vi "Test Process Multiple Stop.vi"(8 "error in (no error)":errorcluster, 11 "Process Test In":refnum<class "Process Dev Test.lvclass">) -> (0 "error out":errorcluster, 3 "Process Test Out":refnum<class "Process Dev Test.lvclass">)   [LabVIEW 2020, in "Process Dev Test.lvclass"]
uses:
  Process Dev Test.lvclass
  C:/Program Files (x86)/National Instruments/LabVIEW 2020/vi.lib/Astemes/LUnit/Test Case.lvclass
  source/Framework Test Suite/Mock Error Handler/Mock Error Handler.lvclass
  C:/Git/astemes-triarc-framework/source/Framework/Error Handler Interface/Error Handler Interface.lvclass
  source/Framework/Process/Process.lvclass/Process.ctl
  <vilib>/Astemes/LUnit/Test Case.lvclass/Test Case.ctl
  <vilib>/Astemes/LUnit/LUnit Assertion Result.lvclass/LUnit Assertion Result.ctl
  <vilib>/Astemes/LUnit/LUnit Test Case Result.lvclass/LUnit Test Case Result.ctl
  <vilib>/Astemes/LUnit/LUnit Method Result.lvclass/LUnit Method Result.ctl
  source/Framework/Process/Protected/Messaging/Enqueue Message.vi
  source/Framework/Process/Public/Lifecycle/Get Lifecycle State.vi
  source/Framework/Process/Private/SubVIs/Wait for finish.vi
  source/Framework/Process/Private/SubVIs/Set Lifecycle State.vi
  <vilib>/Astemes/LUnit/Palette/Pass.vi
  <vilib>/Astemes/LUnit/Palette/Fail.vi
  <vilib>/Astemes/LUnit/Set Assertion Type.vi
  source/Framework/Process/Private/SubVIs/Handle Debug Data.vi
  <vilib>/Utility/error.llb/Clear Errors.vi
  <vilib>/Astemes/LUnit/Add test result.vi
  <vilib>/Astemes/LUnit/LUnit Write Passed.vi
  <vilib>/Astemes/LUnit/LUnit Write Message.vi
  <vilib>/Astemes/LUnit/LUnit Write Description.vi
  <vilib>/Astemes/LUnit/LUnit Write Assertion Type.vi
  source/Framework/Logging/Log Debug.vi
  <vilib>/AdvancedString/1D String Array to Delimited String.vi
  <vilib>/Utility/High Resolution Relative Seconds.vi
  <vilib>/Astemes/LUnit/LUnit Record Assertion Result.vi
  <vilib>/Astemes/LUnit/LUnit Aggregate Assertion Results.vi
  <vilib>/Astemes/LUnit/Assertion Result/LUnit Read Status.vi
  <vilib>/Astemes/LUnit/LUnit Read Message.vi
  <vilib>/Astemes/LUnit/LUnit Read Description.vi
  <vilib>/Astemes/LUnit/Method Result/LUnit Merge Status.vi
  <vilib>/Astemes/LUnit/LUnit Concatenate result strings.vi
  <vilib>/Utility/error.llb/Error Cluster From Error Code.vi
  source/Framework/Process/Public/Read Name.vi
  <vilib>/Astemes/LUnit/LUnit Assertion Result.lvclass
  source/Framework/Process/Process.lvclass
  <vilib>/Astemes/LUnit/Test Case.lvclass
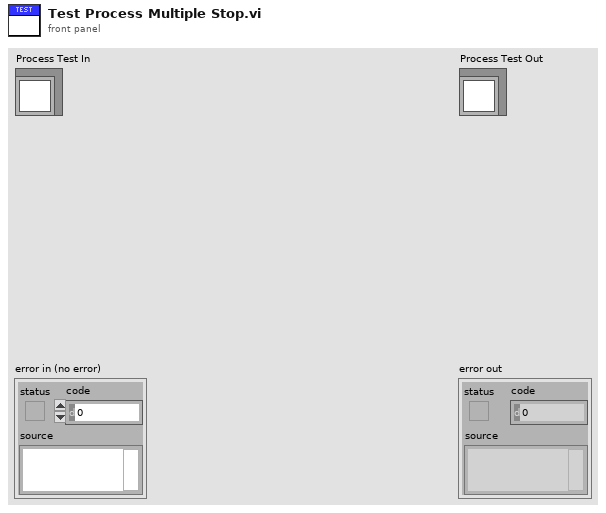
[diagram p1: front panel]
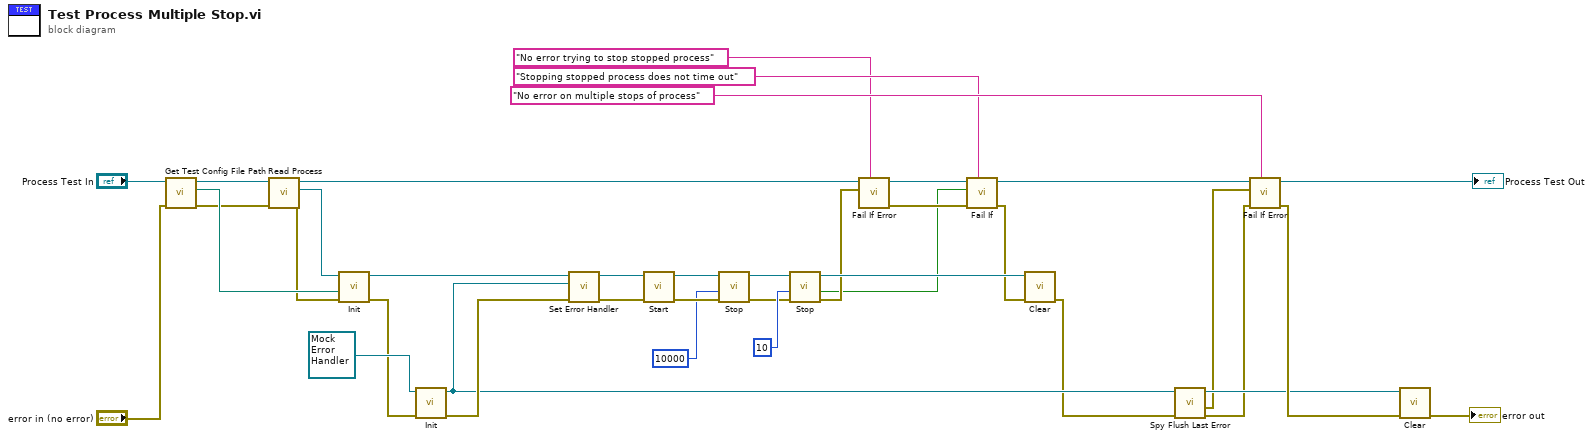
[diagram p0: block diagram]
diagram:
  n1 = call "Get Test Config File Path.vi"("error in (no error)"="error in (no error)", "Process Test In"="Process Test In") -> ("error out"=w29:errorcluster, "Test config path"=w32:path, "Process Test Out"=w34:refnum<class "Process Dev Test.lvclass">)  [unwired: 7 in]
  n2 = call "Read Process.vi"("error in (no error)"=w29, "Process Test in"=w34) -> ("error out"=w30:errorcluster, "Process.lvclass"=w31:refnum<class "Process.lvclass">, "Process Test out"=w10:refnum<class "Process Dev Test.lvclass">)  [unwired: 7 in]
  n3 = call-dynamic "Init.vi"("error in (no error)"=w30, "Config File Path"=w32, "Process In"=w31) -> ("error out"=w20:errorcluster, "Process Out"=w35:refnum<class "Process.lvclass">)  [unwired: 7 in]
  n4 = call-dynamic "Init.vi"("error in (no error)"=w20, "Mock Error Handler In"=refnum<class "Mock Error Handler.lvclass"> refnum ("Mock Error Handler.lvclass")) -> ("error out"=w24:errorcluster, "Mock Error Handler Out"=w23:refnum<class "Mock Error Handler.lvclass">)  [unwired: 8 in]
  n5 = call "Set Error Handler.vi"("error in (no error)"=w24, "Error Handler"=w23, "Process In"=w35) -> ("error out"=w25:errorcluster, "Process Out"=w26:refnum<class "Process.lvclass">)  [unwired: 7 in]
  n6 = call "Start.vi"("error in (no error)"=w25, "Process In"=w26) -> ("error out"=w37:errorcluster, "Process Out"=w38:refnum<class "Process.lvclass">)  [unwired: 7 in, 1 out]
  n7 = call "Stop.vi"("error in (no error)"=w37, "timeout in ms (-1)"=10000, "Process In"=w38) -> ("error out"=w6:errorcluster, "Process Out"=w28:refnum<class "Process.lvclass">)  [unwired: 6 in, 1 out]
  n8 = call "Stop.vi"("error in (no error)"=w6, "timeout in ms (-1)"=10, "Process In"=w28) -> ("error out"=w5:errorcluster, "timed out?"=w3:bool, "Process Out"=w27:refnum<class "Process.lvclass">)  [unwired: 6 in]
  n9 = call <vilib>:"Fail If Error.vi"("Description"="No error trying to stop stopped process", "Assert error"=w5, "LUnit Test Case In"=w10) -> ("error out"=w13:errorcluster, "LUnit Test Case Out"=w14:refnum<class "Process Dev Test.lvclass">)  [unwired: 7 in]
  n10 = call <vilib>:"Fail If.vi"("Description"="Stopping stopped process does not time out", "error in (no error)"=w13, "Fail?"=w3, "LUnit Test Case In"=w14) -> ("error out"=w4:errorcluster, "LUnit Test Case Out"=w9:refnum<class "Process Dev Test.lvclass">)  [unwired: 6 in]
  n11 = call-dynamic "Clear.vi"("error in (no error)"=w4, "Process In"=w27) -> ("error out"=w19:errorcluster)  [unwired: 9 in]
  n12 = call "Spy Flush Last Error.vi"("error in (no error)"=w19, "Mock Error Handler In"=w23) -> ("error out"=w2:errorcluster, "Error"=w1:errorcluster, "Mock Error Handler Out"=w17:refnum<class "Mock Error Handler.lvclass">)  [unwired: 7 in]
  n13 = call <vilib>:"Fail If Error.vi"("Description"="No error on multiple stops of process", "error in (no error)"=w2, "Assert error"=w1, "LUnit Test Case In"=w9) -> ("error out"=w18:errorcluster, "LUnit Test Case Out"=→"Process Test Out":refnum<class "Process Dev Test.lvclass">)  [unwired: 6 in]
  n14 = call-dynamic "Clear.vi"("error in (no error)"=w18, "Mock Process In"=w17) -> ("error out"=→"error out":errorcluster)  [unwired: 9 in]
